vi "Query-Setpoint.vi"(6 "error in (no error)":errorcluster, 7 "Output channel":T1, 8 "VISA resource name":refnum<visa-resource-name>) -> (0 "error out":errorcluster, 3 "Recalled setpoint / V":dbl, 5 "VISA resource name out":refnum<visa-resource-name>)   [LabVIEW 2015, in "YbTempCtrl.lvlib"]
doc: "Get the currently set setpoint"
uses:
  YbTempCtrl.lvlib
  Typedefs/OutputChannelTypedef.ctl
panel:
  out "read buffer":string
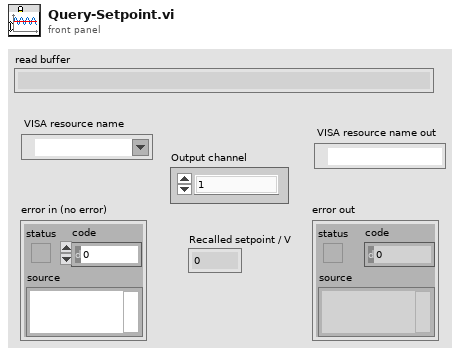
[diagram p1: front panel]
types:
  T1 = typedef "YbTempCtrl.lvlib/OutputChannelTypedef.ctl" = enum16{"1", "2", "3", "4", "BPA", "BPB"}
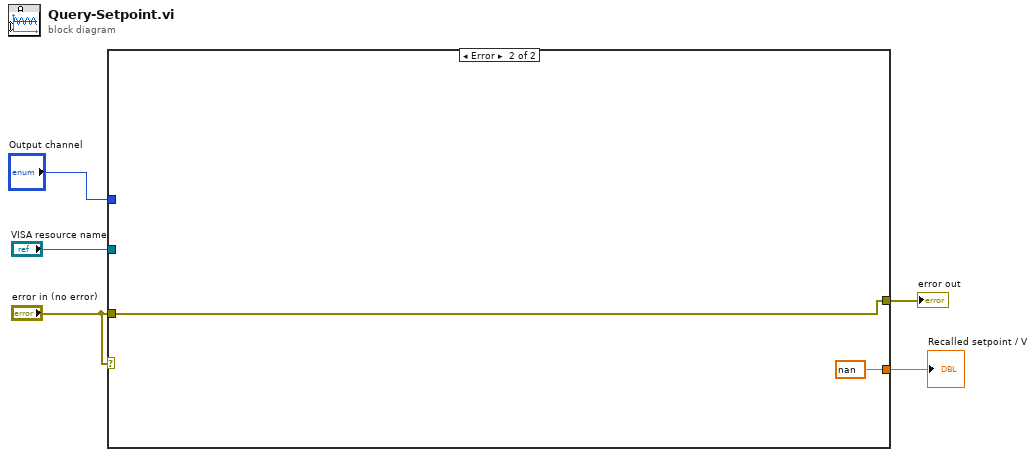
[diagram p0: block diagram]
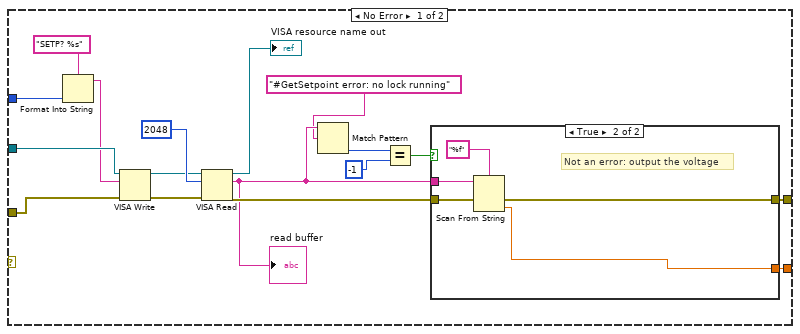
[diagram p2: hidden frame]
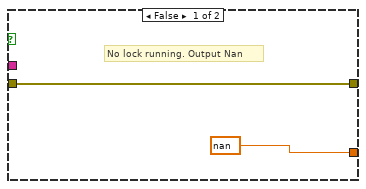
[diagram p3: hidden frame]
diagram:
  n1 = case shown="Error" "error in (no error)" {
    tunnel: "VISA resource name" -> [w22 _]
    tunnel: "error in (no error)" -> [w20 w31]
    tunnel: [w16 w31] -> w4
    tunnel: "Output channel" -> [w12 _]
    tunnel: [w6 nan] -> w2
    frame No Error {
      n2 = Format Into String(format string="SETP? %s" ("write buffer"), w12) -> (resulting string=w15:string)  [unwired: 2 in, 1 out]
      n3 = VISA Write(VISA resource name=w22, write buffer=w15, error in (no error)=w20) -> (VISA resource name out=w14:refnum<visa-resource-name>, error out=w13:errorcluster)  [unwired: 1 out]
      n4 = VISA Read(VISA resource name=w14, byte count=u32 2048, error in (no error)=w13) -> (VISA resource name out=→"VISA resource name out":refnum<visa-resource-name>, read buffer=w11:string, error out=w17:errorcluster)  [unwired: 1 out]
      "read buffer" <- w11
      n5 = Match Pattern(string=w11, regular expression="#GetSetpoint error: no lock running") -> (offset past match=w9:i32)  [unwired: 1 in, 3 out]
      n6 = Equal?(x=w9, y=-1) -> (x = y?=w7:bool)
      n7 = case shown="True" w7 {
        tunnel: w17 -> [w24 w28]
        tunnel: [w24 w27] -> w16
        tunnel: w11 -> [_ w26]
        tunnel: [nan w25] -> w6
        frame False {
          # "No lock running. Output Nan"
        }
        frame True {
          # "Not an error: output the voltage"
          n8 = Scan From String(format string="%f", input string=w26, error in=w28) -> (error out=w27:errorcluster, output 1=w25:dbl)  [unwired: 2 in, 2 out]
        }
      }
    }
    frame Error {
    }
  }
  "error out" <- w4
  "Recalled setpoint / V" <- w2
